vi "SVDFilter.vi"(7 "Input Image":cdb[][](array[numeric]), 9 "Low zero index":i32, 10 "output cluster":T2) -> (2 "Filtered Output":cdb[][][](array[numeric]), 3 "log singular":dbl[](graph))   [LabVIEW 2022 SP3]
uses:
  <vilib>/Analysis/Matrix/Datatypes/ComplexMatrix.ctl
  <vilib>/Analysis/7linalg.llb/Complex Conjugate Transpose Matrix.vi
  <vilib>/Analysis/baseanly.llb/Complex A x B.vi
  <vilib>/Analysis/7linalg.llb/Create Special Complex Matrix.vi
  <vilib>/Analysis/NI_AALPro.lvlib
  <vilib>/Analysis/NI_AALBase.lvlib
  <vilib>/Analysis/Matrix/NI_Matrix.lvlib
panel:
  in  "Filtered Index":i32
  out "Row Cropped data":dbl[][](graph)
  out "log singular 2":dbl[](graph)
  out "Array":dbl[][](array[numeric])
  in  "high zero index":i32
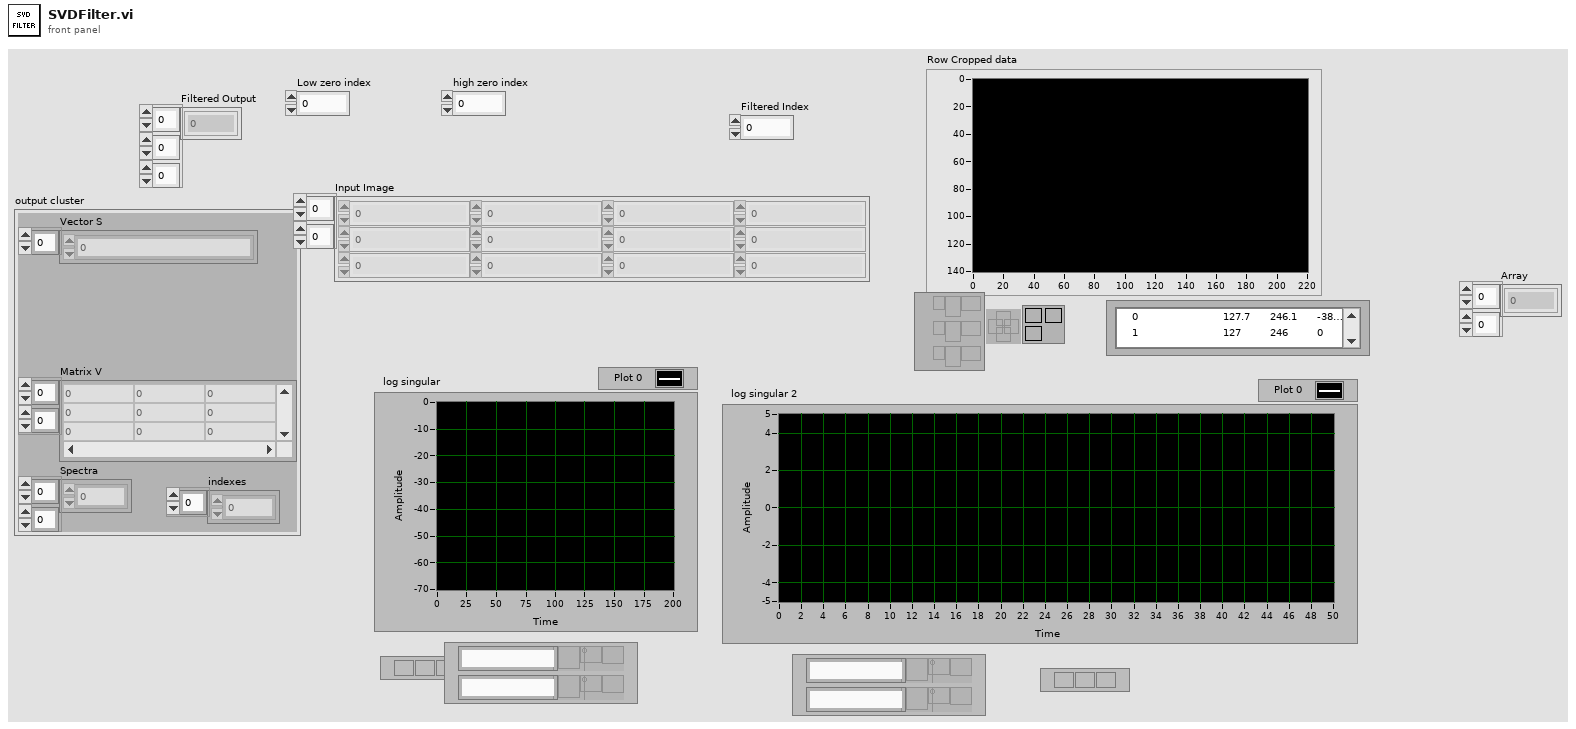
[diagram p1: front panel]
types:
  T1 = typedef "NI_Matrix.lvlib/ComplexMatrix.ctl" = cdb[][]
  T2 = cluster{"Vector S":cdb[], "Matrix V":T1, "Spectra":dbl[][], "indexes":i32[]}
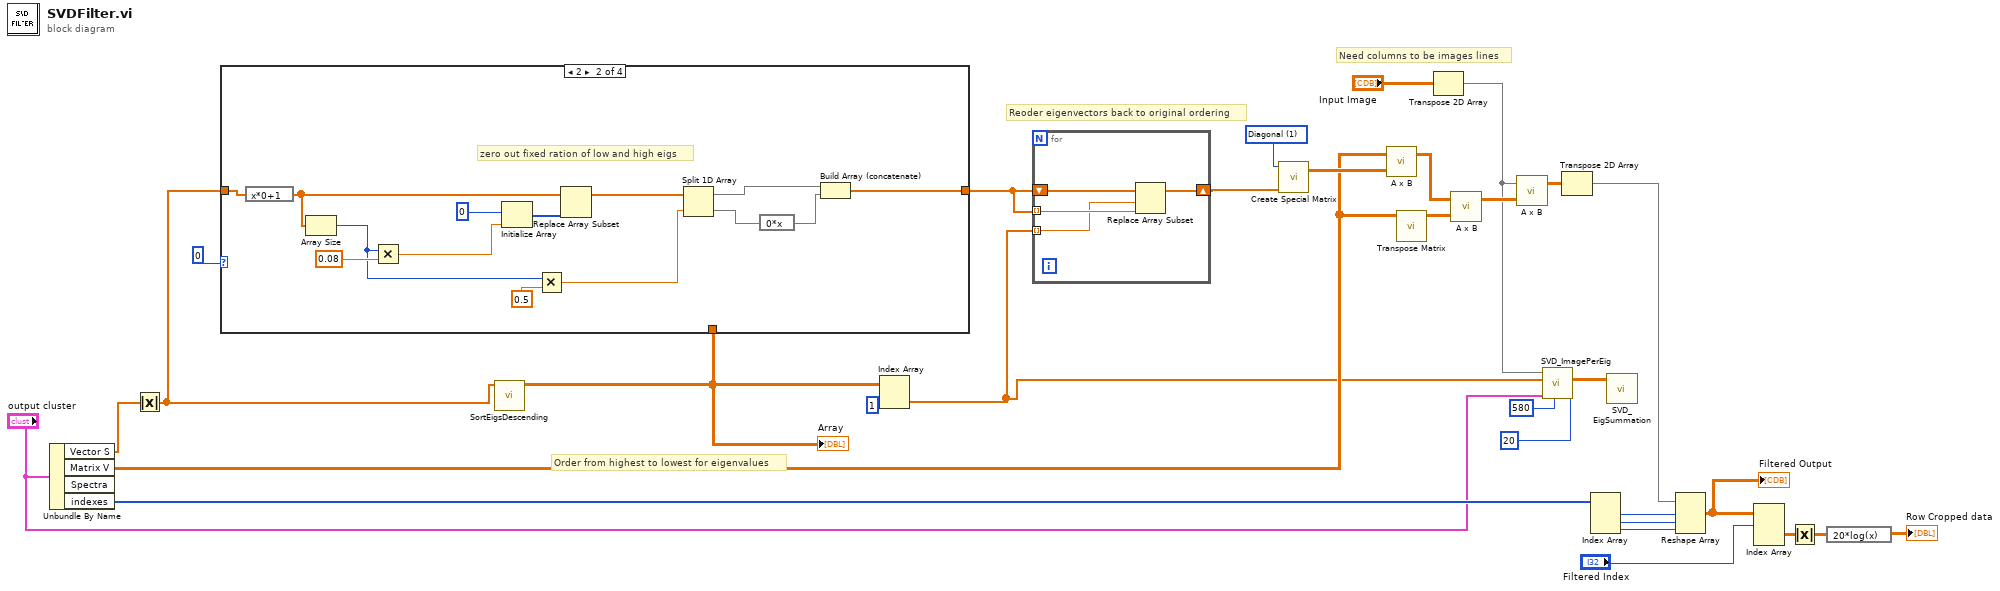
[diagram p0: block diagram]
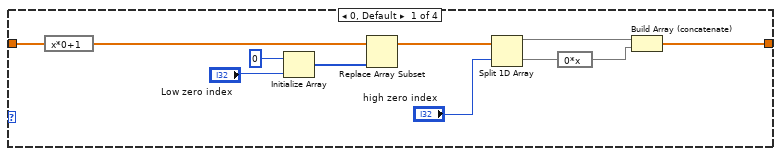
[diagram p2: hidden frame]
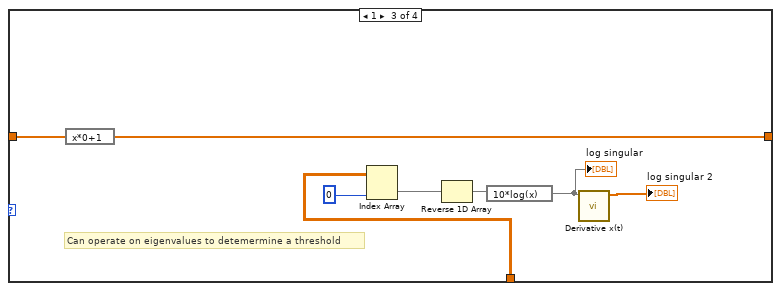
[diagram p3: hidden frame]
diagram:
  w30 = 1 items=["Identity", "Diagonal", "Toeplitz", "Vandermonde", "Companion", "Hankel", "Hadamard", "Wilkinson", "Hilbert", "Inverse Hilbert", "Rosser", "Pascal"] ("matrix type")
  # "Need columns to be images lines"
  # "Reoder eigenvectors back to original ordering"
  # "Order from highest to lowest for eigenvalues"
  n1 = Unbundle By Name("output cluster") -> ("Vector S"=w26:cdb[], "Matrix V"=w27:T1, "indexes"=w23:i32[])  [unwired: 1 out]
  n2 = Absolute Value(x=w26) -> (abs(x)=w7:dbl[])
  n3 = call "SortEigsDescending.vi"("Array in"=w7) -> ("Array out"=w15:dbl[][])  [unwired: 10 in]
  "Array" <- w15
  n4 = case shown="2" 0 {
    tunnel: w7 -> [w35 w52 w59 w65]
    tunnel: [w32 w53 w58 w65] -> w14
    tunnel: w15 -> [_ _ w57 _]
    frame 0, Default {
      n5 = expression code="x*0+1"(w35) -> (w34:dbl[])
      n6 = Initialize Array(0 ("dimension size"), "Low zero index") -> (w37:i32[])
      n7 = Replace Array Subset(array=w34, new element=w37) -> (w40:dbl[])  [unwired: 1 in]
      n8 = Split 1D Array(array=w40, index="high zero index") -> (first subarray=w41:dbl[], second subarray=w33:dbl[])
      n9 = expression code="0*x"(w33) -> (w42:dbl[])
      n10 = Build Array (concatenate)(w41, w42) -> (w32:dbl[])
    }
    frame 2 {
      # "zero out fixed ration of low and high eigs"
      n11 = expression code="x*0+1"(w52) -> (w50:dbl[])
      n12 = Array Size(array=w50) -> (size(s)=w48:i32)
      n13 = Multiply(x=w48, y=0.08) -> (x*y=w44:dbl)
      n14 = Initialize Array(0 ("dimension size"), w44) -> (w43:i32[])
      n15 = Multiply(x=w48, y=0.5) -> (x*y=w46:dbl)
      n16 = Replace Array Subset(array=w50, new element=w43) -> (w54:dbl[])  [unwired: 1 in]
      n17 = Split 1D Array(array=w54, index=w46) -> (first subarray=w55:dbl[], second subarray=w51:dbl[])
      n18 = expression code="0*x"(w51) -> (w56:dbl[])
      n19 = Build Array (concatenate)(w55, w56) -> (w53:dbl[])
    }
    frame 1 {
      # "Can operate on eigenvalues to detemermine a threshold"
      n20 = expression code="x*0+1"(w59) -> (w58:dbl[])
      n21 = Index Array(array=w57, index (col)=0 ("disabled index (col)")) -> (element=w63:dbl[])  [unwired: 1 in]
      n22 = Reverse 1D Array(array=w63) -> (reversed array=w62:dbl[])
      n23 = expression code="10*log(x)"(w62) -> (w61:dbl[])
      "log singular" <- w61
      n24 = call <vilib>:"Derivative x(t).vi"("X"=w61) -> ("dX/dt"=→"log singular 2":dbl[])  [unwired: 9 in, 1 out]
    }
    frame 3 {
      # "leave alone"
    }
  }
  n25 = Index Array(array=w15, index (col)=1 ("disabled index (col)")) -> (element=w3:dbl[])  [unwired: 1 in]
  n26 = for {
    tunnel: w3 -> [w66] mode=indexing
    shift-right: [w68] -> w12
    shift-left: w14 -> [w69]
    tunnel: w14 -> [w67] mode=indexing
    n27 = Replace Array Subset(array=w69, new element=w67, index=w66) -> (w68:dbl[])
  }
  n28 = call-poly <vilib>:"Create Special Matrix.vi"("matrix type"=w30, "Input Vector1"=w12) -> ("Special Matrix"=w29:T1)  [unwired: 3 in, 1 out]
  n29 = call-poly <vilib>:"A x B.vi"("B"=w29, "A"=w27) -> ("A x B"=w31:T1)  [unwired: 1 out]
  n30 = call-poly <vilib>:"Transpose Matrix.vi"("Input Matrix"=w27) -> ("Matrix Conjugate Transpose"=w28:T1)  [unwired: 9 in, 1 out]
  n31 = Transpose 2D Array(2D array="Input Image") -> (transposed array=w6:cdb[][])
  n32 = call-poly <vilib>:"A x B.vi"("B"=w28, "A"=w31) -> ("A x B"=w10:T1)  [unwired: 1 out]
  n33 = call-poly <vilib>:"A x B.vi"("B"=w10, "A"=w6) -> ("A x B"=w9:T1)  [unwired: 1 out]
  n34 = call "SVD_ImagePerEig.vi"("frame"=20, "first N index"=580, "output cluster"="output cluster", "Index Order"=w3, "Input Casarati"=w6) -> ("StackedImages"=w4:cdb[][][])  [unwired: 6 in]
  n35 = Transpose 2D Array(2D array=w9) -> (transposed array=w8:T1)
  n36 = Index Array(array=w23) -> (element #1=w22:i32, element #2=w21:i32, element #3=w20:i32)  [unwired: 3 in]
  n37 = call "SVD_EigSummation.vi"("Stacked Images"=w4) -> ()  [unwired: 11 in]
  n38 = Reshape Array(w8, w22, w21, w20) -> (w16:cdb[][][])
  "Filtered Output" <- w16
  n39 = Index Array(array=w16, index (dim 0)="Filtered Index") -> (element=w19:cdb[][])  [unwired: 2 in]
  n40 = Absolute Value ("Absolute Value.vi")(x=w19) -> (abs(x)=w25:dbl[][])
  n41 = expression code="20*log(x)"(w25) -> (→"Row Cropped data":dbl[][])
